vi "Read Setting.vi"(8 "error in (no error)":errorcluster, 11 "Update Bool Array in":refnum<class "Update Bool Array.lvclass">) -> (0 "error out":errorcluster, 2 "Setting":bool[](array[boolean]), 3 "Update Bool Array out":refnum<class "Update Bool Array.lvclass">)   [LabVIEW 2014, in "Update Bool Array.lvclass"]
uses:
  Update Bool Array.lvclass
  Update Bool Array.lvclass/Update Bool Array.ctl
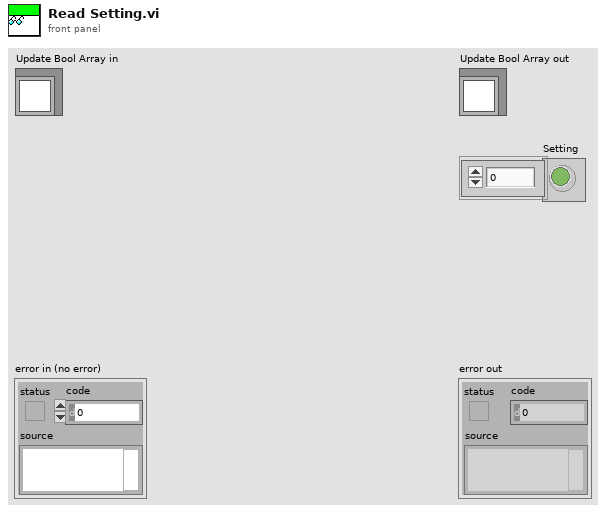
[diagram p1: front panel]
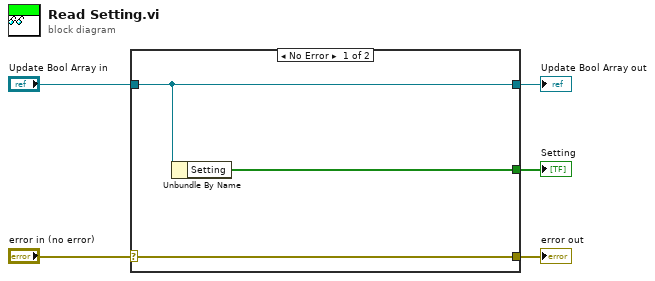
[diagram p0: block diagram]
diagram:
  n1 = case shown="No Error" "error in (no error)" {
    selector: "error in (no error)" -> [w8 w9]
    tunnel: [w8 w9] -> w4
    tunnel: [w7 w10] -> w2
    tunnel: "Update Bool Array in" -> [w7 w10]
    tunnel: [w6 _] -> w1
    frame No Error {
      n2 = Unbundle By Name(w7) -> ("Setting"=w6:bool[])
    }
    frame Error {
    }
  }
  "error out" <- w4
  "Update Bool Array out" <- w2
  "Setting" <- w1
